vi "Read Image Text.vi"(8 "Error In":errorcluster, 10 "ROI Descriptor":T2 {"Contours"."Type" items=["No Selection", "Point", "Line", "Rectangle", "Oval", "Polygon", "Freehand Region", "Annulus", "Unused2", "Unused3", "Broken Line", "Freehand Line", "Rotated Rectangle"]}, 11 "Image Ref":T1) -> (0 "Error Out":errorcluster, 3 "Line of Text":string)   [LabVIEW 2018, in "Receipt Parsing.lvlib"]
uses:
  Receipt Parsing.lvlib
  <vilib>/vision/Image Controls.llb/IMAQ Image.ctl
  Action.ctl
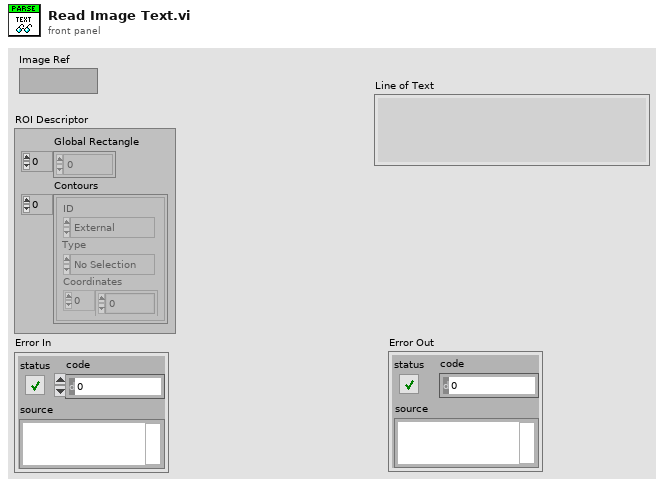
[diagram p1: front panel]
types:
  T1 = typedef "IMAQ Image.ctl" = refnum<image>
  T2 = typedef "ROI Descriptor" = cluster{"Global Rectangle":i32[], "Contours":cluster{"ID":enum32{"External", "Internal"}, "Type":u32, "Coordinates":i32[]}[]}
  T3 = typedef "Receipt Parsing.lvlib/Action.ctl" = enum16{"Init", "Read Image Text", "Close"}
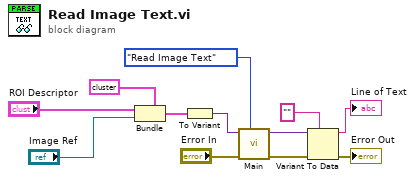
[diagram p0: block diagram]
diagram:
  n1 = Bundle(cluster=cluster{"ROI Descriptor":T2, "Image Out":T1} {"ROI Descriptor"={"Global Rectangle"=[], "Contours"=[]}, "Image Out"=refnum}, "ROI Descriptor"="ROI Descriptor", "Image Out"="Image Ref") -> (w5:cluster{"ROI Descriptor":T2, "Image Out":T1})
  n2 = To Variant(anything=w5) -> (Variant=w1:variant)
  n3 = call "Main.vi"("Action"=Action."Read Image Text", "Error In"="Error In", "Data In"=w1) -> ("Error Out"=w10:errorcluster, "Data Out"=w11:variant)  [unwired: 7 in]
  n4 = Variant To Data(error in=w10, type="", Variant=w11) -> (data=→"Line of Text":string, error out=→"Error Out":errorcluster)
